vi "Add Step To Front.vi"(6 "Step Name":string, 8 "error in (no error)":errorcluster, 9 "Reply Channel":refnum<notifier>, 10 "Parameter":variant, 11 "Actor in":refnum<class "Actor.lvclass">) -> (0 "error out":errorcluster)   [LabVIEW 2020, in "Actor.lvclass"]
uses:
  Actor.lvclass
  Sequencer/Sequencer.lvclass
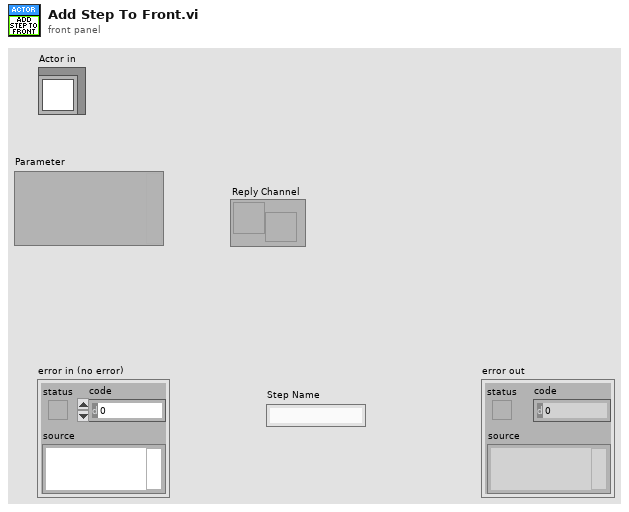
[diagram p1: front panel]
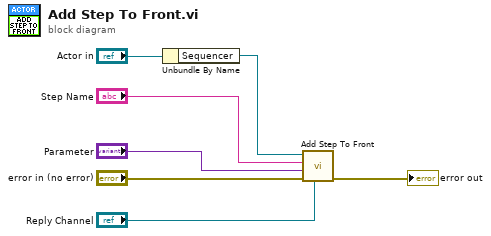
[diagram p0: block diagram]
diagram:
  n1 = Unbundle By Name("Actor in") -> ("Sequencer"=w4:refnum<class "Sequencer.lvclass">)
  n2 = call "Add Step To Front.vi"("Reply Channel"="Reply Channel", "error in (no error)"="error in (no error)", "Parameter"="Parameter", "Step Name"="Step Name", "Sequencer in"=w4) -> ("error out"=→"error out":errorcluster)  [unwired: 6 in]
